vi "Timer.vi"(6 "Action":T1=enum."TimeElapsed", 11 "Limit":dbl) -> (1 "Over limit?":bool, 3 "Elapsed Time":dbl)   [LabVIEW 2020]
uses:
  #typedef_TimerAction.ctl
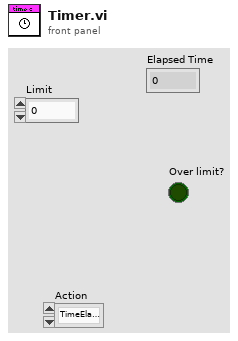
[diagram p1: front panel]
types:
  T1 = typedef "#typedef_TimerAction.ctl" = enum16{"Reset", "TimeElapsed"}
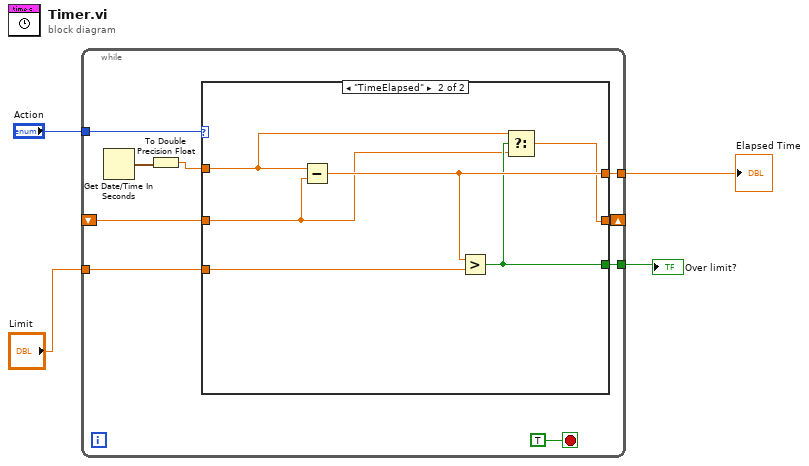
[diagram p0: block diagram]
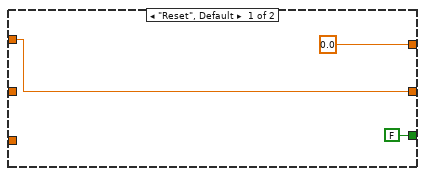
[diagram p2: hidden frame]
diagram:
  n1 = while {
    tunnel: "Action" -> [w12]
    shift-right: [w8] -> _
    shift-left: _ -> [w9]
    tunnel: [w7] -> w3
    tunnel: [w6] -> w2
    tunnel: "Limit" -> [w5]
    stop <- TRUE stop-if-true
    n2 = Get Date/Time In Seconds() -> (seconds since 1Jan1904=w11:timestamp)
    n3 = To Double Precision Float(number=w11) -> (double precision float=w10:dbl)
    n4 = case shown="\"TimeElapsed\"" w12 {
      tunnel: w10 -> [w16 w18]
      tunnel: w9 -> [_ w17]
      tunnel: [0.0 w22] -> w7
      tunnel: [w16 w19] -> w8
      tunnel: [FALSE w20] -> w6
      tunnel: w5 -> [_ w21]
      frame "Reset", Default {
      }
      frame "TimeElapsed" {
        n5 = Subtract(x=w18, y=w17) -> (x-y=w22:dbl)
        n6 = Greater?(x=w22, y=w21) -> (0:w20:bool)
        n7 = Select(t=w18, s=w20, f=w17) -> (s? t:f=w19:dbl)
      }
    }
  }
  "Elapsed Time" <- w3
  "Over limit?" <- w2
